vi "Camber controller May 4 2016.vi"() -> ()   [LabVIEW 2014]
uses:
  <vilib>/Instr/_visa.llb/VISA Configure Serial Port (Instr).vi
  <vilib>/Utility/file.llb/Write To Spreadsheet File (string).vi
  <vilib>/Utility/file.llb/Read From Spreadsheet File (string).vi
  Environmental Chamber LabVIEW and Instruments/Drivers and Software/keithley_6430/Keithley 6430/Public/Data/Read (Single Point).vi
  Environmental Chamber LabVIEW and Instruments/Drivers and Software/LabVIEW 8.2 Drivers/keithley_24xx/Keithley 24XX/Public/Data/Read (Single Point).vi
  Environmental Chamber LabVIEW and Instruments/Drivers and Software/keithley_24xx/Keithley 24XX/Keithley 24XX.lvlib
  Environmental Chamber LabVIEW and Instruments/Drivers and Software/keithley_6430/Keithley 6430/Keithley 6430.lvlib
panel:
  in  "Sample names 2":T1={"QCM1 sample"="aQCM2", "QCM2 sample"="aQCM2", "QCM3 sample"="aQCM3", "QCM4 sample"="aQCM4", "QCM5 sample"="aQCM5", "QCM6 sample"="aQCM6", "SRS sample"="sample_SRS", "K-2420 sample"="Keithley2420", "K-6430 sample"="Keithley6430", "K-2100 sample"="Keithley6430"}
  out "pressure chart":cluster{"pressure":dbl}(graph)
  out "K-6430 (Ohm)":cluster{"Measurement":dbl}(graph)
  out "K-2420 (Ohm)":cluster{"Resistance":sgl}(graph)
  in  "Data saving options":T2={"Save during sequence only"=TRUE, "Save now"=FALSE, "Stop program when sequence ends"=TRUE, "Delay between data points (s)"=0.0, "Experiment Notes"="", "Currently saving data"=FALSE, "Data file save path"=path ""} {"Delay between data points (s)" min=0.0 max=30.0 format="%#_13g"}
  out "Temp (C)":dbl
  in  "Set pressure parameters":T3={"valve % open"=100.0, "Desired pressure"=0.0, "Vapor sccm"=0.0, "Gas sccm"=0.0, "Valve"=enum."% Open", "Pressure Mode"=enum."Abs. pressure", "analyte partial pressure"=100.0} {"analyte partial pressure" min=0.0 max=100.0 step=5.0; "Gas sccm" min=0 max=200 step=5; "Vapor sccm" min=0 max=200 step=5; "Desired pressure" min=0.0 max=760.0 step=5.0; "valve % open" min=0.0 max=100.0 step=5.0 format="%#_2f"}
  out "Actual":T4 {"actual gas flow" format="%#_3g"; "Actual vapor flow" format="%#_3g"; "actual pressure" format="%#_3g"; "Valve position (%)" format="%#_2f"}
  out "arduino QCM plots":T5
  out "QCM Freq. (MHz)":T6 {"QCM1" format="%#_8g"; "QCM2" format="%#_8g"; "QCM3" format="%#_8g"; "QCM4" format="%#_8g"; "QCM5" format="%#_8g"; "QCM6" format="%#_8g"}
  out "Sequence\npreview":cluster{dbl[], dbl[]}[](graph)
  in  "Gate time":u16(ring)=1 items=["0.1 seconds", "1.0 seconds", "10.0 seconds"]
  out "MHz":dbl format="%.6f"
  out "QCM plot":T7(graph)
  in  "User-defined\nsequence":string[][](table) caption="Create sequence"
  out "Sequence end time":string
  in  "Run Sequence":bool
  in  "Import sequence file":bool
  in  "Save sequence":bool
  in  "Clear sequence":bool
  in  "Turbo pump\nauto on":bool=TRUE caption="Turbo pump auto on"
  out "Start Time":string
  in  "stop":bool
  in  "Clear all charts":bool
  out "appended array":dbl[](array[numeric]) caption="atm\nTorr"
  in  "rapidox O2 Sensor":bool
  in  "setnag O2 Pump":bool
  in  "Baud Rate 2":i32(ring)=2 items=["2400", "4800", "9600", "19200", "38400", "57600", "115200"]
  in  "Com Port":i32(ring) items=["Com 1", "Com 2", "Com 3", "Com 4", "Com 5", "Com 6", "COM 7", "COM 8", "COM 9", "COM 10", "COM 11", "COM 12", "com 13", "COM 14"]
  in  "Com Port 2":i32(ring) items=["Com 1", "Com 2", "Com 3", "Com 4", "Com 5", "Com 6", "COM 7", "COM 8", "COM 9", "COM 10", "COM 11", "COM 12", "com 13", "COM 14"]
  out "Waveform Chart":cluster{dbl}(graph)
  out "O2 Concentration (PPM)":dbl
  out "Waveform Chart 6":cluster{dbl}(graph)
  # "Pressure Control"
  # "Gas/Vapor Sequence"
  # "SRS QCM"
  # "Currently Unused"
  # "100%"
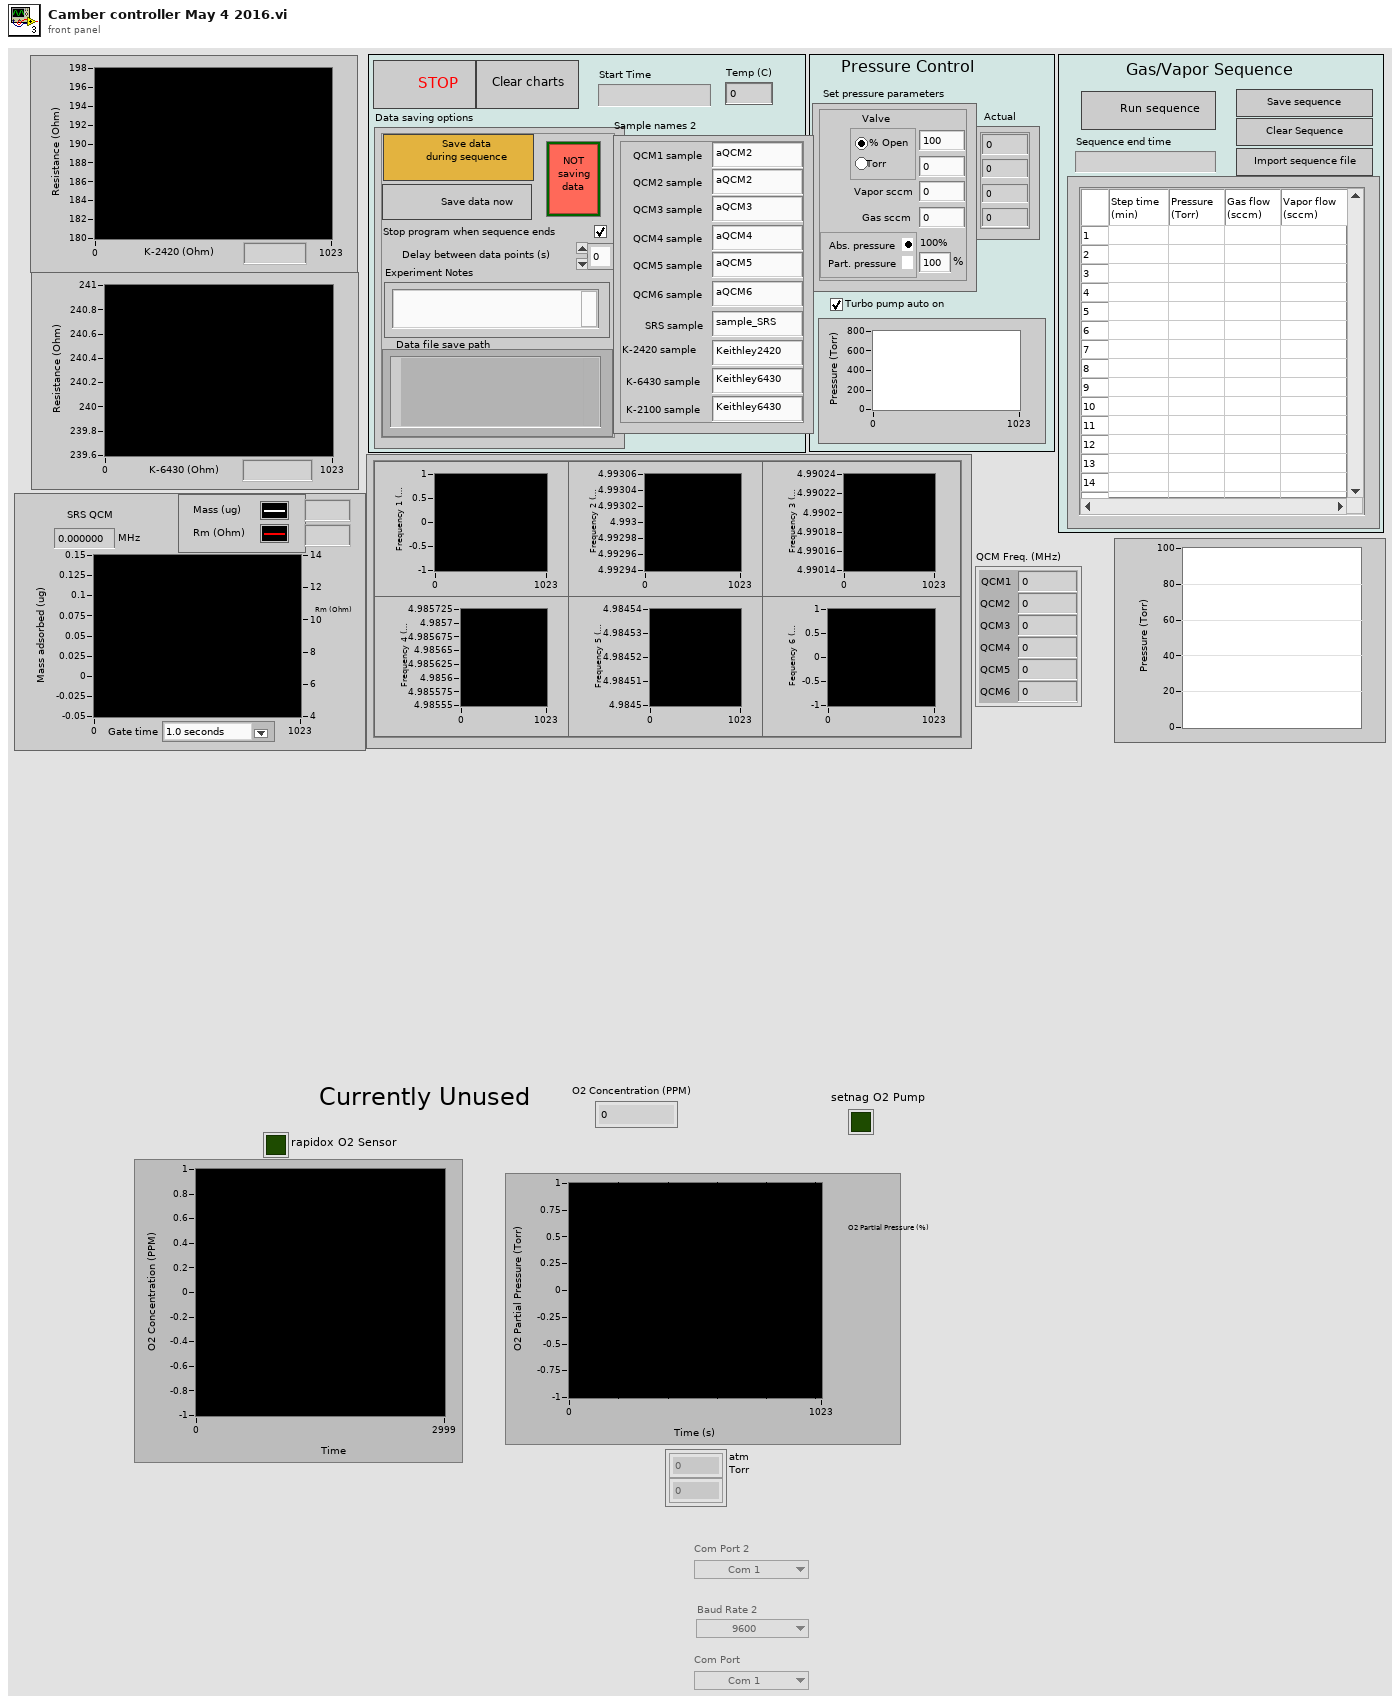
[diagram p1: front panel]
types:
  T1 = cluster{"QCM1 sample":string, "QCM2 sample":string, "QCM3 sample":string, "QCM4 sample":string, "QCM5 sample":string, "QCM6 sample":string, "SRS sample":string, "K-2420 sample":string, "K-6430 sample":string, "K-2100 sample":string}
  T2 = cluster{"Save during sequence only":bool, "Save now":bool, "Stop program when sequence ends":bool, "Delay between data points (s)":dbl, "Experiment Notes":string, "Currently saving data":bool, "Data file save path":path}
  T3 = cluster{"valve % open":dbl, "Desired pressure":dbl, "Vapor sccm":sgl, "Gas sccm":sgl, "Valve":enum32{"% Open", "Torr "}, "Pressure Mode":enum32{"Abs. pressure", " Part. pressure"}, "analyte partial pressure":dbl}
  T4 = cluster{"Valve position (%)":dbl, "actual pressure":dbl, "Actual vapor flow":dbl, "actual gas flow":dbl}
  T5 = cluster{"arduino qcm 1":dbl, "arduino qcm 2":dbl, "arduino qcm 3":dbl, "arduino qcm 4":dbl, "arduino qcm 5":dbl, "arduino qcm 6":dbl}
  T6 = cluster{"QCM1":dbl, "QCM2":dbl, "QCM3":dbl, "QCM4":dbl, "QCM5":dbl, "QCM6":dbl}
  T7 = cluster{"Numeric Control":dbl, "Resistance out":dbl}
  T8 = enum16{"open", "open or create", "create or replace", "create", "open (read only)"}
  T9 = enum16{"no parity", "odd parity", "even parity", "mark parity", "space parity"}
  T10 = enum8{"Enabled", "Disabled", "Disabled and Grayed Out"}
  T11 = cluster{"task out":refnum<k21>, "error out":errorcluster, "task out":refnum<k21>, "error out":errorcluster, "task out":refnum<k21>, "error out":errorcluster, "VISA resource name":refnum<visa-resource-name>, "error out":errorcluster}
  T12 = cluster{"task out":refnum<k21>, "error out":errorcluster, "task out":refnum<k21>, "error out":errorcluster, "task out":refnum<k21>, "error out":errorcluster, "VISA resource name out":refnum<visa-resource-name>, "error out":errorcluster}
  T13 = cluster{bool, "VISA resource name":refnum<visa-resource-name>, "error out":errorcluster}
  T14 = cluster{bool, "VISA resource name out":refnum<visa-resource-name>, "error out":errorcluster}
  T15 = cluster{"Arduino 1":refnum<visa-resource-name>, "Arduino 2":refnum<visa-resource-name>, "Arduino 3":refnum<visa-resource-name>, "Arduino 4":refnum<visa-resource-name>, "Arduino 5":refnum<visa-resource-name>, "Arduino 6":refnum<visa-resource-name>}
  T16 = cluster{"VISA resource name out":refnum<visa-resource-name>, "error out":errorcluster, "VISA resource name out":refnum<visa-resource-name>, "error out":errorcluster, "VISA resource name out":refnum<visa-resource-name>, "error out":errorcluster, "VISA resource name out":refnum<visa-resource-name>, "error out":errorcluster, "VISA resource name out":refnum<visa-resource-name>, "error out":errorcluster, "VISA resource name out":refnum<visa-resource-name>, "error out":errorcluster}
  T17 = cluster{"f":dbl, "f":dbl, "f":dbl, "f":dbl, "f":dbl, "f":dbl}
  T18 = cluster{"String":string, "String":string, "String":string}
  T19 = cluster{"Boolean":bool, "VISA resource name out":refnum<visa-resource-name>, "error out":errorcluster}
  T20 = cluster{bool, "Turbo pump\nauto on":bool, "current  step # out":i32}
  T21 = cluster{"Present (s)":dbl, "Run Sequence":bool, "Set pressure parameters":cluster{"valve % open":dbl, "Desired pressure":dbl, "Vapor sccm":sgl, "Gas sccm":sgl, "Valve":enum32{"% Open", "Torr "}, "Pressure Mode":enum32{"Abs. pressure", " Part. pressure"}, "analyte partial pressure":dbl}, "sequence end time":timestamp}
  T22 = cluster{"VISA Refnum out":refnum<visa-resource-name>, "error out":errorcluster, "VISA Refnum out":refnum<visa-resource-name>, "error out":errorcluster, "VISA Refnum out":refnum<visa-resource-name>, "error out":errorcluster, "VISA Refnum out":refnum<visa-resource-name>, "error out":errorcluster, "VISA Refnum out":refnum<visa-resource-name>, "error out":errorcluster, "VISA Refnum out":refnum<visa-resource-name>, "error out":errorcluster}
  T23 = cluster{"f":string, "f":string, "f":string, "f":string, "f":string, "f":string}
  T24 = cluster{bool, "VISA out":refnum<visa-resource-name>, "error out":errorcluster}
  T25 = cluster{"Boolean":bool, "VISA out":refnum<visa-resource-name>, "error out":errorcluster}
  T26 = cluster{"User-defined\nsequence":refnum<vi>, "Sequence end time":refnum<vi>, "Run Sequence":refnum<vi>}
  T27 = cluster{"pressure":string, "RH":string, "gas flow":string, "vapor flow":string}
  T28 = cluster{"Valve position (%)":dbl, "pressure":dbl, "vapor flow":dbl, "gas flow":dbl}
  T29 = cluster{"task out":refnum<k21>, "error out":errorcluster, "task out":refnum<k21>, "error out":errorcluster, "task out":refnum<k21>, "error out":errorcluster, "VISA Refnum out":refnum<visa-resource-name>, "error out":errorcluster}
  T30 = cluster{"sequence on?":bool, "sequence end time":timestamp, "current  step # out":i32}
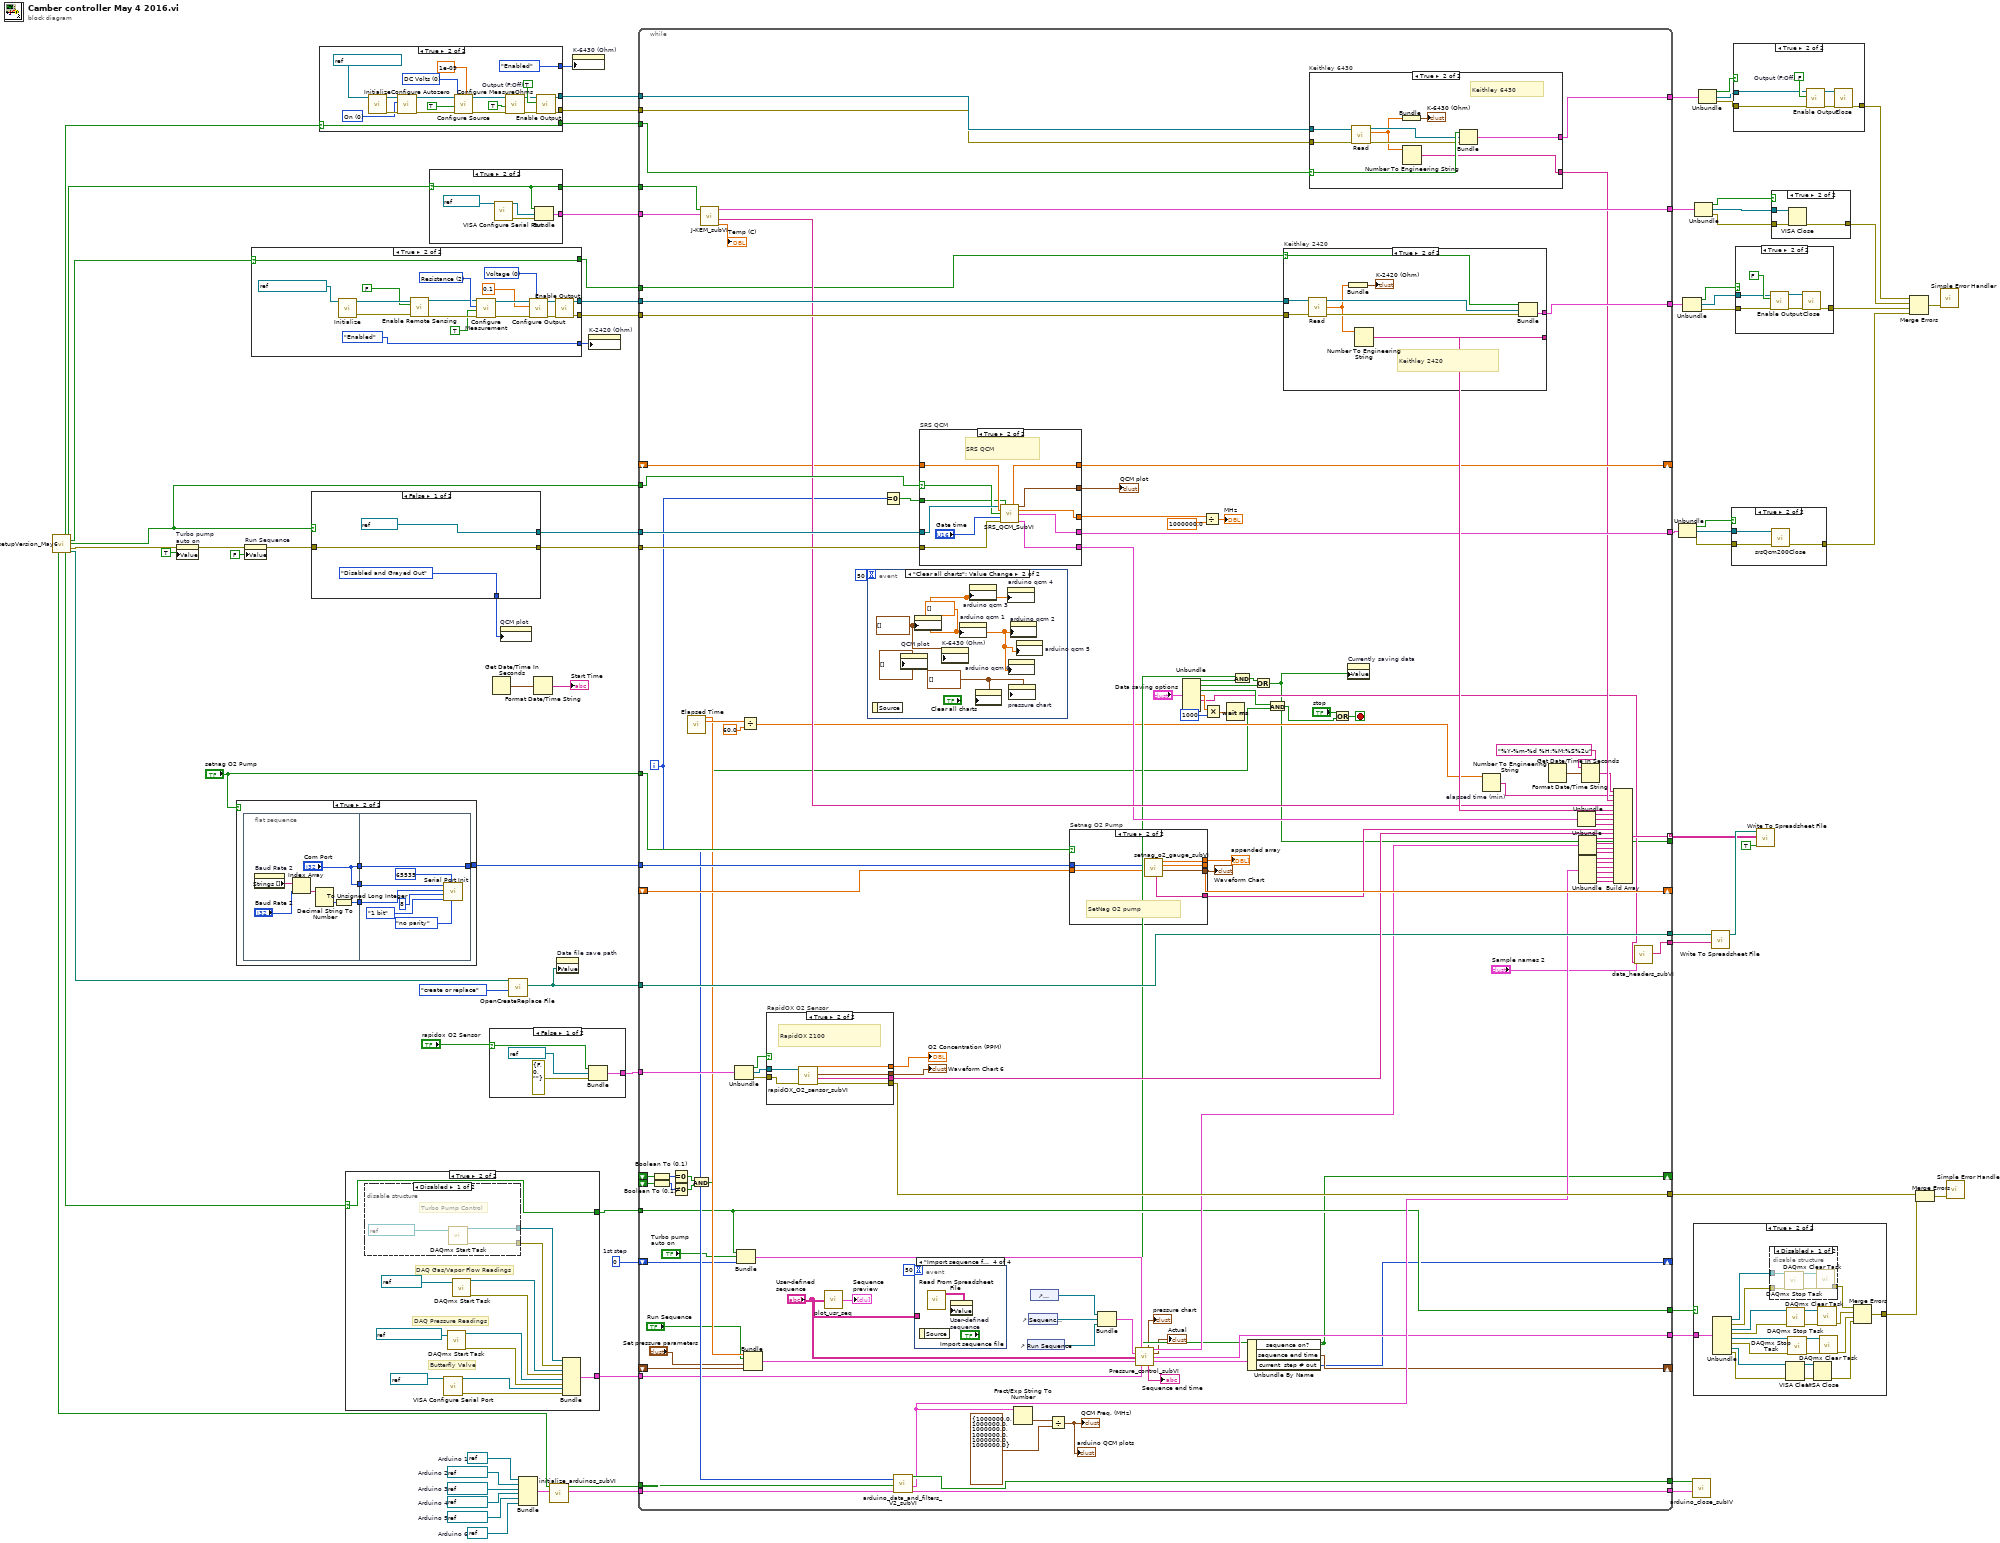
[diagram p0: block diagram]
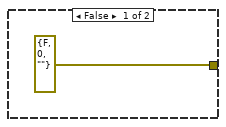
[diagram p2: hidden frame]
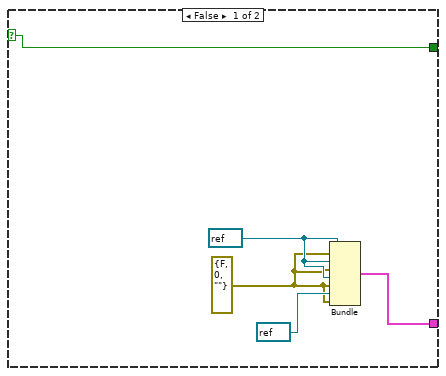
[diagram p4: hidden frame]
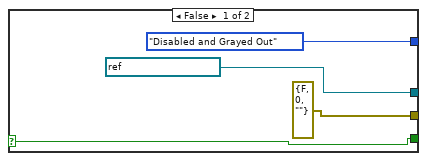
[diagram p7: hidden frame]
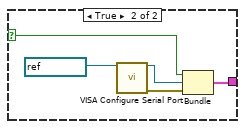
[diagram p8: hidden frame]
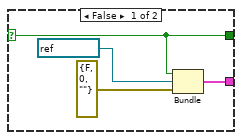
[diagram p10: hidden frame]
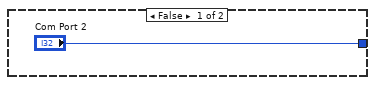
[diagram p11: hidden frame]
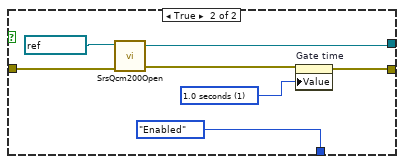
[diagram p13: hidden frame]
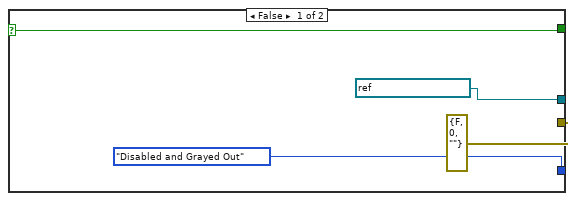
[diagram p15: hidden frame]
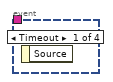
[diagram p16: hidden frame]
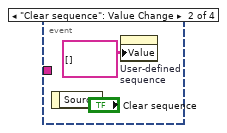
[diagram p17: hidden frame]
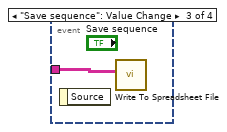
[diagram p18: hidden frame]
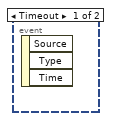
[diagram p19: hidden frame]
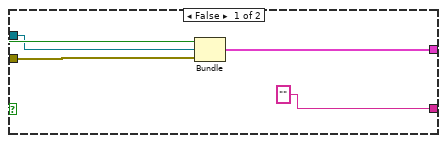
[diagram p20: hidden frame]
diagram:
  w17 = refnum<visa-resource-name> refnum  # Arduino 6
  w18 = refnum<visa-resource-name> "COM51"  # Arduino 5
  w19 = refnum<visa-resource-name> "COM50"  # Arduino 4
  w20 = refnum<visa-resource-name> "COM49"  # Arduino 3
  w21 = refnum<visa-resource-name> "COM48"  # Arduino 2
  w10 = refnum<visa-resource-name> refnum  # Arduino 1
  w37 = 0  # 1st step
  n1 = call "setupVersion_May6.vi"() -> ("Keithley 6431"=w27:bool, "J-KEM2"=w26:bool, "Keithley 2421"=w6:bool, "SRS QCM 2"=w30:bool, "error IO"=w2:errorcluster, "Arduino2"=w15:bool, "Pressure control 2"=w28:bool, "Save file path 2"=w29:path)  [unwired: 8 in]
  n2 = property on="Turbo pump\nauto on" class="Bool (strict)"(error in=w2, "Value"=TRUE ("Turbo\npump")) -> (error out=w33:errorcluster)  [unwired: 1 in, 1 out]
  n3 = case shown="True" "setnag O2 Pump" {
    tunnel: ["Com Port 2" w80] -> w72
    frame False {
    }
    frame True {
      n4 = flat-sequence {
        tunnel: ["Com Port"] -> w83
        tunnel: [w85] -> w82
        tunnel: ["Com Port"] -> w81
        tunnel: w83 -> [w91]
        tunnel: w82 -> [w90]
        tunnel: w81 -> [w92]
        tunnel: [w92] -> w80
        frame #0 {
          n5 = property on="Baud Rate 2" class="Ring (strict)"() -> ("Strings []"=w87:string[])  [unwired: 2 in, 2 out]
          n6 = Index Array(array=w87, index="Baud Rate 2") -> (element=w88:string)
          n7 = Decimal String To Number(string=w88) -> (number=w86:i32)  [unwired: 2 in, 1 out]
          n8 = To Unsigned Long Integer(number=w86) -> (unsigned 32bit integer=w85:u32)
        }
        frame #1 {
          n9 = call <vilib>:"Serial Port Init.vi"("parity"=T9."no parity", "buffer size"=u16 65535, "stop bits"=enum16{"1 bit", "1.5 bits", "2 bits"}."1 bit", "data bits"=u16 8, "baud rate"=w90, "port number"=w91) -> ()  [unwired: 1 in, 1 out]
        }
      }
    }
  }
  n10 = property on="Run Sequence" class="Bool (strict)"(error in=w33, "Value"=FALSE ("Run Sequence")) -> (error out=w35:errorcluster)  [unwired: 1 in, 1 out]
  n11 = case shown="True" w6 {
    selector: w6 -> [w97 w101]
    tunnel: [refnum<visa-resource-name> "GPIB1::24::INSTR" ("VISA resource name") w110] -> w76
    tunnel: [errorcluster {"status"=FALSE, "code"=0, "source"=""} ("error out") w105] -> w75
    tunnel: [T10."Disabled and Grayed Out" ("Disabled") T10."Enabled" ("Disabled")] -> w24
    tunnel: [w97 w101] -> w5
    frame False {
    }
    frame True {
      w112 = u16 0 items=["Voltage", "Current"] ("Source Mode  (0: Voltage)")
      w117 = u16 2 items=["Volts", "Current", "Resistance"] ("Function (0: Volts)")
      n12 = call "Initialize.vi"("VISA resource name"=refnum<visa-resource-name> "GPIB1::24::INSTR") -> ("error out"=w106:errorcluster, "VISA resource name out"=w109:refnum<visa-resource-name>)  [unwired: 9 in]
      n13 = call "Enable Remote Sensing.vi"("error in (no error)"=w106, "Enable Remote Sensing (T: Enable)"=FALSE ("4-wire?"), "VISA resource name"=w109) -> ("error out"=w107:errorcluster, "VISA resource name out"=w108:refnum<visa-resource-name>)  [unwired: 7 in]
      n14 = call "Configure Measurement.vi"("error in (no error)"=w107, "Enable Auto Range (T:Enable)"=TRUE, "Function (0: Volts)"=w117, "VISA resource name"=w108) -> ("error out"=w116:errorcluster, "VISA resource name out"=w115:refnum<visa-resource-name>)  [unwired: 6 in]
      n15 = call "Configure Output.vi"("Source Mode  (0: Voltage)"=w112, "error in (no error)"=w116, "Output Level (0)"=0.1 ("Applied Voltage (V)"), "VISA resource name"=w115) -> ("error out"=w114:errorcluster, "VISA resource name out"=w113:refnum<visa-resource-name>)  [unwired: 6 in]
      n16 = call "Enable Output.vi"("error in (no error)"=w114, "VISA resource name"=w113) -> ("error out"=w105:errorcluster, "VISA resource name out"=w110:refnum<visa-resource-name>)  [unwired: 8 in]
    }
  }
  n17 = case shown="False" w30 {
    tunnel: [refnum<visa-resource-name> "COM6" ("VISA in") w125] -> w74
    tunnel: [w120 w122] -> w73
    tunnel: w35 -> [w120 w127]
    tunnel: [T10."Disabled and Grayed Out" ("Disabled") T10."Enabled" ("Disabled")] -> w25
    frame False {
    }
    frame True {
      w124 = u16 1 items=["0.1 seconds", "1.0 seconds", "10.0 seconds"] ("Gate time")
      n18 = call "SrsQcm200Open.vi"("error in"=w127, "VISA in"=refnum<visa-resource-name> "COM6") -> ("error out"=w123:errorcluster, "VISA out"=w125:refnum<visa-resource-name>)  [unwired: 3 in]
      n19 = property on="Gate time" class="Ring (strict)"(error in=w123, "Value"=w124) -> (error out=w122:errorcluster)  [unwired: 1 in, 1 out]
    }
  }
  n20 = case shown="True" w27 {
    selector: w27 -> [w129 w133]
    tunnel: [refnum<visa-resource-name> "GPIB0::29::INSTR" ("VISA resource name") w146] -> w44
    tunnel: [errorcluster {"status"=FALSE, "code"=0, "source"=""} ("error out") w147] -> w43
    tunnel: [T10."Disabled and Grayed Out" ("Disabled") T10."Enabled" ("Disabled")] -> w23
    tunnel: [w129 w133] -> w4
    frame False {
    }
    frame True {
      w135 = u16 0 items=["DC Volts", "DC Current"] ("Source Function (0: DC Volts)")
      w142 = u16 0 items=["On", "Off", "Once"] ("Autozero  (0: On)")
      w150 = TRUE  # Output (F:Off)
      n21 = call "Initialize.vi"("VISA resource name"=refnum<visa-resource-name> "GPIB0::30::INSTR") -> ("error out"=w143:errorcluster, "VISA resource name out"=w144:refnum<visa-resource-name>)  [unwired: 4 in, 5 out]
      n22 = call "Configure Autozero.vi"("error in (no error)"=w143, "Autozero  (0: On)"=w142, "VISA resource name"=w144) -> ("error out"=w138:errorcluster, "VISA resource name out"=w140:refnum<visa-resource-name>)  [unwired: 7 in]
      n23 = call "Configure Source.vi"("I-Source Level [A]"=1e-09, "error in (no error)"=w138, "Auto Range (T:Enable)"=TRUE, "Source Function (0: DC Volts)"=w135, "VISA resource name"=w140) -> ("error out"=w137:errorcluster, "VISA resource name out"=w139:refnum<visa-resource-name>)  [unwired: 5 in]
      n24 = call "Configure MeasureOhms.vi"("error in (no error)"=w137, "Auto Range (T:Enable)"=TRUE, "VISA resource name"=w139) -> ("error out"=w151:errorcluster, "VISA resource name out"=w149:refnum<visa-resource-name>)  [unwired: 3 in, 4 out]
      n25 = call "Enable Output.vi"("error in (no error)"=w151, "Enable Output (F:Off)"=w150, "VISA resource name"=w149) -> ("error out"=w147:errorcluster, "VISA resource name out"=w146:refnum<visa-resource-name>)  [unwired: 7 out]
    }
  }
  n26 = case shown="True" w28 {
    selector: w28 -> [w152 w157]
    tunnel: [w153 w159] -> w38
    tunnel: [w152 w157] -> w3
    frame False {
      w155 = refnum<k21> refnum ("task out")
      w154 = errorcluster {"status"=FALSE, "code"=0, "source"=""} ("error out")
      n27 = Bundle("task out"=w155, "error out"=w154, "task out"=w155, "error out"=w154, "task out"=w155, "error out"=w154, "VISA resource name"=refnum<visa-resource-name> refnum, "error out"=w154) -> (w153:T11)  [unwired: 1 in]
    }
    frame True {
      # "DAQ Gas/Vapor Flow Readings"
      # "DAQ Pressure Readings"
      # "Butterfly Valve"
      n28 = disable-structure shown="Disabled" {
        disable-tunnel: [w171 _] -> w166
        disable-tunnel: [w170 _] -> w165
        frame Disabled {
          # "Turbo Pump Control"
          n29 = call <vilib>:"DAQmx Start Task.vi"("task/channels in"=refnum<k21> "TurboON") -> ("task out"=w171:refnum<k21>, "error out"=w170:errorcluster)  [unwired: 13 in]
        }
        frame Enabled {
        }
      }
      n30 = call-poly "VISA Configure Serial Port"("VISA resource name"=refnum<visa-resource-name> "COM5") -> ("VISA resource name out"=w160:refnum<visa-resource-name>, "error out"=w158:errorcluster)  [unwired: 13 in]
      n31 = call <vilib>:"DAQmx Start Task.vi"("task/channels in"=refnum<k21> "AllDaqReadings") -> ("task out"=w162:refnum<k21>, "error out"=w161:errorcluster)  [unwired: 13 in]
      n32 = call <vilib>:"DAQmx Start Task.vi"("task/channels in"=refnum<k21> "Setflow") -> ("task out"=w164:refnum<k21>, "error out"=w163:errorcluster)  [unwired: 13 in]
      n33 = Bundle("task out"=w166, "error out"=w165, "task out"=w164, "error out"=w163, "task out"=w162, "error out"=w161, "VISA resource name out"=w160, "error out"=w158) -> (w159:T12)  [unwired: 1 in]
    }
  }
  n34 = case shown="True" w26 {
    selector: w26 -> [w173 w178]
    tunnel: [w174 w179] -> w61
    tunnel: [w173 w178] -> w55
    frame False {
      n35 = Bundle(w173, "VISA resource name"=refnum<visa-resource-name> "COM3", "error out"=errorcluster {"status"=FALSE, "code"=0, "source"=""}) -> (w174:T13)  [unwired: 1 in]
    }
    frame True {
      n36 = call-poly "VISA Configure Serial Port"("VISA resource name"=refnum<visa-resource-name> "COM3") -> ("VISA resource name out"=w180:refnum<visa-resource-name>, "error out"=w177:errorcluster)  [unwired: 13 in]
      n37 = Bundle(w178, "VISA resource name out"=w180, "error out"=w177) -> (w179:T14)  [unwired: 1 in]
    }
  }
  n38 = case shown="False" "rapidox O2 Sensor" {
    selector: "rapidox O2 Sensor" -> [w182 w187]
    tunnel: [w183 w188] -> w51
    frame False {
      n39 = Bundle(w182, "VISA resource name"=refnum<visa-resource-name> "COM7", "error out"=errorcluster {"status"=FALSE, "code"=0, "source"=""}) -> (w183:T13)  [unwired: 1 in]
    }
    frame True {
      n40 = call-poly "VISA Configure Serial Port"("VISA resource name"=refnum<visa-resource-name> "COM7") -> ("VISA resource name out"=w189:refnum<visa-resource-name>, "error out"=w186:errorcluster)  [unwired: 13 in]
      n41 = Bundle(w187, "VISA resource name out"=w189, "error out"=w186) -> (w188:T14)  [unwired: 1 in]
    }
  }
  n42 = Get Date/Time In Seconds() -> (seconds since 1Jan1904=w78:timestamp)
  n43 = property on="QCM plot" class="WFChart (strict)"("DisabledEnum"=w25) -> ()  [unwired: 2 in, 2 out]
  n44 = call "OpenCreateReplace File.vi"("function (open:0)"=T8."create or replace", "file path"=w29) -> ("new file path"=w1:path)  [unwired: 6 in, 3 out]
  n45 = Bundle("Arduino 1"=w10, "Arduino 2"=w21, "Arduino 3"=w20, "Arduino 4"=w19, "Arduino 5"=w18, "Arduino 6"=w17) -> (w9:T15)  [unwired: 1 in]
  n46 = Format Date/Time String(seconds (now)=w78) -> (date/time string=→"Start Time":string)  [unwired: 2 in]
  n47 = call "initialize_arduinos_subVI.vi"("arduino 1-6 addresses"=w9, "arduinos on?"=w15) -> ("arduino 1-6 address and errors"=w14:T16, "arduinos on/off"=w16:bool)  [unwired: 8 in]
  n48 = property on="Data file save path" class="Path"("Value"=w1) -> ()  [unwired: 2 in, 2 out]
  n49 = property on="K-6430 (Ohm)" class="WFChart (strict)"("DisabledEnum"=w23) -> ()  [unwired: 2 in, 2 out]
  n50 = property on="K-2420 (Ohm)" class="WFChart (strict)"("DisabledEnum"=w24) -> ()  [unwired: 2 in, 2 out]
  n51 = while {
    shift-right: [w311] -> _
    shift-left: _ -> [w310]
    tunnel: [w281] -> w22 mode=indexing if=w192
    tunnel: w5 -> [w287]
    tunnel: w76 -> [w309]
    tunnel: w75 -> [w308]
    tunnel: w74 -> [w307]
    tunnel: w73 -> [w306]
    tunnel: w30 -> [w305]
    tunnel: "setnag O2 Pump" -> [w299]
    tunnel: w72 -> [w304]
    tunnel: [w301] -> w69
    tunnel: [w300] -> w65
    tunnel: w61 -> [w298]
    tunnel: [w297] -> w60
    tunnel: w55 -> [w295]
    tunnel: w51 -> [w293]
    tunnel: [w288] -> w31
    tunnel: [w286] -> w50
    tunnel: w1 -> [w286]
    shift-right: [w279] -> _
    shift-left: _ -> [w280]
    tunnel: w44 -> [w285]
    tunnel: w43 -> [w284]
    tunnel: [w283] -> w42
    tunnel: w3 -> [w223]
    tunnel: [w223] -> w39
    tunnel: w38 -> [w217]
    shift-right: [w219] -> _
    shift-left: w37 -> [w225]
    tunnel: [w192] -> _
    shift-right: [w220] -> _
    shift-left: _ -> [w234]
    tunnel: w16 -> [w263]
    tunnel: w14 -> [w262]
    tunnel: [w261] -> w12
    tunnel: [w260] -> w13
    tunnel: [w251] -> w11
    tunnel: [w237] -> w8
    tunnel: w4 -> [w236]
    shift-right: [w203] -> _
    shift-left: _ -> [w215]
    shift-left: _ -> [w214]
    i -> [w264]
    stop <- w199 stop-if-true
    n52 = Boolean To (0,1)(Boolean=w215) -> (0, 1=w213:i16)
    n53 = Boolean To (0,1)(Boolean=w214) -> (0, 1=w212:i16)
    n54 = Equal To 0?(x=w213) -> (x = 0?=w210:bool)
    n55 = Not Equal To 0?(x=w212) -> (x != 0?=w211:bool)
    n56 = call "Elapsed Time"() -> ("Present (s)"=w244:dbl, "Elapsed Time (s)"=w277:dbl)  [unwired: 12 in, 6 out]
    n57 = And(x=w210, y=w211) -> (x .and. y?=w197:bool)
    n58 = call "J-KEM_subVI.vi"("Address in"=w298, "J-KEM on?"=w295) -> ("Temp (C)"=→"Temp (C)":dbl, "String data out"=w296:string, "Address out"=w297:T19)  [unwired: 6 in, 1 out]
    n59 = Unbundle(w293) -> (w292:bool, "VISA resource name out"=w291:refnum<visa-resource-name>, "error out"=w290:errorcluster)
    n60 = Bundle(w223, "Turbo pump\nauto on"="Turbo pump\nauto on", "current  step # out"=w225) -> (w222:T20)  [unwired: 1 in]
    n61 = Divide(x=w277, y=60.0) -> (x/y=w201:dbl)
    n62 = Bundle("Present (s)"=w244, "Run Sequence"="Run Sequence", "Set pressure parameters"="Set pressure parameters", "sequence end time"=w234) -> (w216:T21)  [unwired: 1 in]
    n63 = case "RapidOX O2 Sensor" shown="True" w292 {
      tunnel: w291 -> [_ w343]
      tunnel: w290 -> [w336 w342]
      tunnel: ["" w341] -> w289
      tunnel: [w336 w340] -> w288
      tunnel: [0.0 w339] -> w276
      tunnel: [cluster{dbl} {0.0} w338] -> w275
      frame False {
      }
      frame True {
        # "RapidOX 2100"
        n64 = call "rapidOX_O2_sensor_subVI.vi"("error in (no error)"=w342, "VISA Refnum in"=w343) -> ("error out"=w340:errorcluster, "String"=w341:string, "Cluster"=w338:cluster{"Numeric Control":dbl}, "Numeric Control"=w339:dbl)  [unwired: 6 in]
      }
    }
    "O2 Concentration (PPM)" <- w276
    "Waveform Chart 6" <- w275
    n65 = call "plot_usr_seq.vi"("User-defined sequence"="User-defined\nsequence") -> ("Sequence Preview"=→"Sequence\npreview":cluster{dbl[], dbl[]}[])
    n66 = event shown="[1] \"Clear all charts\": Value Change" {
      selector: _ -> [_ _]
      dyn-events: _ -> [_ _]
      timeout: 50 -> [_ _]
      event Timeout {
        n67 = event-data() -> ()  [unwired: 1 in, 3 out]
      }
      event "Clear all charts": Value Change {
        w316 = cluster{dbl}[] [] ("History Data")
        w318 = cluster{"Resistance":sgl}[] [] ("History Data")
        w317 = dbl[] [] ("History Data")
        n68 = event-data() -> ()  [unwired: 1 in, 1 out]
        n69 = property on="QCM plot" class="WFChart (strict)"("History Data"=cluster{dbl, "Resistance out":dbl}[] []) -> ()  [unwired: 2 in, 2 out]
        n70 = property on="K-2420 (Ohm)" class="WFChart (strict)"("History Data"=w318) -> ()  [unwired: 2 in, 2 out]
        n71 = property on="K-6430 (Ohm)" class="WFChart (strict)"("History Data"=w318) -> ()  [unwired: 2 in, 2 out]
        n72 = property on="arduino qcm 1" class="WFChart (strict)"("History Data"=w317) -> ()  [unwired: 2 in, 2 out]
        n73 = property on="arduino qcm 3" class="WFChart (strict)"("History Data"=w317) -> ()  [unwired: 2 in, 2 out]
        n74 = property on="Waveform Chart" class="WFChart (strict)"("History Data"=w316) -> ()  [unwired: 2 in, 2 out]
        n75 = property on="arduino qcm 4" class="WFChart (strict)"("History Data"=w317) -> ()  [unwired: 2 in, 2 out]
        n76 = property on="arduino qcm 6" class="WFChart (strict)"("History Data"=w317) -> ()  [unwired: 2 in, 2 out]
        n77 = property on="pressure chart" class="WFChart (strict)"("History Data"=w316) -> ()  [unwired: 2 in, 2 out]
        n78 = property on="arduino qcm 2" class="WFChart (strict)"("History Data"=w317) -> ()  [unwired: 2 in, 2 out]
        n79 = property on="arduino qcm 5" class="WFChart (strict)"("History Data"=w317) -> ()  [unwired: 2 in, 2 out]
      }
    }
    n80 = Equal To 0?(x=w264) -> (x = 0?=w270:bool)
    n81 = call "arduino_data_and_filters_V2_subVI.vi"("loop iteration number"=w264, "arduino 1-6 address and errors"=w262, "arduinos on?"=w263) -> ("arduino 1-6 addresses and errors out"=w260:T22, "arduino 1-6 data out"=w259:T23, "arduinos on? output"=w261:bool)  [unwired: 6 in]
    n82 = event shown="[3] \"Import sequence file\": Value Change" {
      selector: _ -> [_ _ _ _]
      dyn-events: _ -> [_ _ _ _]
      timeout: 50 -> [_ _ _ _]
      tunnel: "User-defined\nsequence" -> [_ _ w314 _]
      event Timeout {
        n83 = event-data() -> ()  [unwired: 1 in, 1 out]
      }
      event "Clear sequence": Value Change {
        n84 = event-data() -> ()  [unwired: 1 in, 1 out]
        n85 = property on="User-defined\nsequence" class="Tbl (strict)"("Value"=string[][] []) -> ()  [unwired: 2 in, 2 out]
      }
      event "Save sequence": Value Change {
        n86 = event-data() -> ()  [unwired: 1 in, 1 out]
        n87 = call-poly <vilib>:"Write To Spreadsheet File.vi"("2D data"=w314) -> ()  [unwired: 7 in, 1 out]
      }
      event "Import sequence file": Value Change {
        n88 = event-data() -> ()  [unwired: 1 in, 1 out]
        n89 = call-poly <vilib>:"Read From Spreadsheet File.vi"() -> ("all rows"=w315:string[][])  [unwired: 7 in, 4 out]
        n90 = property on="User-defined\nsequence" class="Tbl (strict)"("Value"=w315) -> ()  [unwired: 2 in, 2 out]
      }
    }
    n91 = case "SRS QCM" shown="True" w305 {
      selector: w305 -> [w361 w367]
      tunnel: w307 -> [w364 w371]
      tunnel: w306 -> [w363 w372]
      tunnel: [w362 w375] -> w300
      tunnel: w280 -> [_ w374]
      tunnel: [w359 w373] -> w279
      tunnel: [T7 {"Numeric Control"=0.0, "Resistance out"=0.0} ("Cluster") w369] -> w274
      tunnel: [w359 w368] -> w250
      tunnel: w270 -> [_ w366]
      tunnel: [T18 {"String"="", "String"="", "String"=""} ("M,F,MR output cluster") w365] -> w258
      frame False {
        w359 = 0.0
        n92 = Bundle(w361, "VISA out"=w364, "error out"=w363) -> (w362:T24)  [unwired: 1 in]
      }
      frame True {
        # "SRS QCM"
        n93 = call "SRS_QCM_SubVI.vi"("VISA Refnum in"=w371, "first iteration?"=w366, "Frequency out 3"=w374, "Boolean 2"=w367, "Gate time"="Gate time", "error in (no error)"=w372) -> ("Frequency out 2"=w373:dbl, "Cluster"=w369:T7, "Frequency out"=w368:dbl, "Cluster 2"=w375:T25, "M,F,MR output cluster"=w365:T18)  [unwired: 2 in, 3 out]
      }
    }
    "QCM plot" <- w274
    n94 = Fract/Exp String To Number(string=w259) -> (number=w247:T17)  [unwired: 3 in, 1 out]
    n95 = control-ref of="Run Sequence"() -> (w227:refnum<vi>)
    n96 = control-ref of="Sequence end time"() -> (w228:refnum<vi>)
    n97 = control-ref of="User-defined\nsequence"() -> (w229:refnum<vi>)
    n98 = Divide(x=w247, y=T17 {"f"=1000000.0, "f"=1000000.0, "f"=1000000.0, "f"=1000000.0, "f"=1000000.0, "f"=1000000.0}) -> (x/y=→"QCM Freq. (MHz)" →"arduino QCM plots":T17)
    n99 = case "Setnag O2 Pump" shown="True" w299 {
      tunnel: [w379 w384] -> w311
      tunnel: w310 -> [w379 w385]
      tunnel: w304 -> [_ w383]
      tunnel: ["" w382] -> w303
      tunnel: [dbl[] [] w381] -> w273
      tunnel: [cluster{dbl} {0.0} w380] -> w272
      frame False {
      }
      frame True {
        # "SetNag O2 pump"
        n100 = call "setnag_o2_gauge_subVI.vi"("Numeric Control 3"=w385, "Com Port"=w383) -> ("Cluster"=w380:cluster{"Numeric Control":dbl}, "Numeric Control out"=w384:dbl, "Array"=w381:dbl[], "String"=w382:string)  [unwired: 6 in]
      }
    }
    "appended array" <- w273
    "Waveform Chart" <- w272
    n101 = Bundle("User-defined\nsequence"=w229, "Sequence end time"=w228, "Run Sequence"=w227) -> (w226:T26)  [unwired: 1 in]
    n102 = call "Pressure_control_subVI.vi"("press control on / turb pump on / step #"=w222, "references in"=w226, "User-defined\nsequence"="User-defined\nsequence", "output cluster"=w216, "DAQ IDs in"=w217) -> ("pressure"=→"pressure chart":cluster{"pressure":dbl}, "press/RH/gas/vapor"=w242:T27, "pressure params out"=→"Actual":T28, "DAQ IDs out"=w237:T29, "seq on/timestamp/step#"=w221:T30, "date/time string"=→"Sequence end time":string)  [unwired: 5 in]
    n103 = Unbundle("Data saving options") -> ("Save during sequence only"=w204:bool, "Save now"=w207:bool, "Stop program when sequence ends"=w198:bool, "Delay between data points (s)"=w205:dbl, "Experiment Notes"=w195:string)  [unwired: 2 out]
    n104 = Divide(x=w250, y=1000000.0) -> (x/y=→"MHz":dbl)
    n105 = Multiply(x=w205, y=u32 1000 ("x")) -> (x*y=w271:dbl)
    n106 = Wait (ms)(milliseconds to wait=w271) -> ()  [unwired: 1 out]
    n107 = Unbundle By Name(w221) -> ("sequence on?"=w203:bool, "sequence end time"=w220:timestamp, "current  step # out"=w219:i32)
    n108 = And(x=w203, y=w204) -> (x .and. y?=w202:bool)
    n109 = Or(x=w202, y=w207) -> (x .or. y?=w192:bool)
    n110 = And(x=w198, y=w197) -> (x .and. y?=w196:bool)
    n111 = case "Keithley 2420" shown="True" w287 {
      selector: w287 -> [w347 w355]
      tunnel: w309 -> [w346 w350]
      tunnel: w308 -> [w345 w349]
      tunnel: [w344 w353] -> w301
      tunnel: ["" w352] -> w302
      frame False {
        n112 = Bundle(w347, "VISA resource name out"=w346, "error out"=w345) -> (w344:T14)  [unwired: 1 in]
      }
      frame True {
        # "Keithley 2420"
        n113 = call-poly "Read.vi"("VISA resource name"=w350, "error in (no error)"=w349) -> ("VISA resource name out"=w356:refnum<visa-resource-name>, "Resistance"=w351:sgl, "error out"=w354:errorcluster)  [unwired: 7 in, 4 out]
        n114 = Bundle("Resistance"=w351) -> (→"K-2420 (Ohm)":cluster{"Resistance":sgl})  [unwired: 1 in]
        n115 = Number To Engineering String(4:w351) -> (0:w352:string)  [unwired: 3 in]
        n116 = Bundle(w355, "VISA resource name out"=w356, "error out"=w354) -> (w353:T14)  [unwired: 1 in]
      }
    }
    n117 = case "Keithley 6430" shown="True" w236 {
      selector: w236 -> [w323 w333]
      tunnel: w285 -> [w322 w330]
      tunnel: w284 -> [w321 w329]
      tunnel: ["" w332] -> w278
      tunnel: [w320 w331] -> w283
      frame False {
        n118 = Bundle(w323, "VISA resource name out"=w322, "error out"=w321) -> (w320:T14)  [unwired: 1 in]
      }
      frame True {
        # "Keithley 6430"
        n119 = call-poly "Read.vi"("error in (no error)"=w329, "VISA resource name"=w330) -> ("error out"=w328:errorcluster, "Measurement"=w326:dbl, "VISA resource name out"=w327:refnum<visa-resource-name>)  [unwired: 1 in, 6 out]
        n120 = Bundle("Measurement"=w326) -> (→"K-6430 (Ohm)":cluster{"Measurement":dbl})  [unwired: 1 in]
        n121 = Number To Engineering String(4:w326) -> (0:w332:string)  [unwired: 3 in]
        n122 = Bundle(w333, "VISA resource name out"=w327, "error out"=w328) -> (w331:T14)  [unwired: 1 in]
      }
    }
    n123 = Or(x="stop", y=w196) -> (x .or. y?=w199:bool)
    n124 = property on="Currently saving data" class="Bool (strict)"("Value"=w192) -> ()  [unwired: 2 in, 2 out]
    n125 = Number To Engineering String "elapsed time (min)"(4:w201) -> (0:w208:string)  [unwired: 3 in]
    n126 = Get Date/Time In Seconds() -> (seconds since 1Jan1904=w312:timestamp)
    n127 = Unbundle(w258) -> ("String"=w268:string, "String"=w267:string, "String"=w266:string)
    n128 = Unbundle(w242) -> ("pressure"=w241:string, "RH"=w240:string, "gas flow"=w239:string, "vapor flow"=w238:string)
    n129 = Unbundle ("arduino 1-6")(w259) -> ("f"=w257:string, "f"=w256:string, "f"=w255:string, "f"=w254:string, "f"=w253:string, "f"=w252:string)
    n130 = Format Date/Time String(time format string (%c)="%Y-%m-%d %H:%M:%S%2u", seconds (now)=w312) -> (date/time string=w265:string)  [unwired: 1 in]
    n131 = Build Array(w265, w208, w278, w296, w302, w268, w267, w266, w303, w289, w241, w240, w239, w238, w257, w256, w255, w254, w253, w252) -> (w281:string[])
    n132 = call "data_headers_subVI.vi"("Experiment Notes"=w195, "Sample names"="Sample names 2") -> ("data headers"=w251:string[])  [unwired: 9 in]
  }
  n133 = Unbundle(w65) -> ("Boolean"=w64:bool, "VISA out"=w63:refnum<visa-resource-name>, "error out"=w62:errorcluster)
  n134 = Unbundle(w69) -> (w68:bool, "VISA resource name out"=w67:refnum<visa-resource-name>, "error out"=w66:errorcluster)
  n135 = call "arduino_close_subIV.vi"("arduino 1-6 addresses and errors out"=w13, "arduinos on?"=w12) -> ()  [unwired: 10 in]
  n136 = case shown="True" w39 {
    tunnel: w8 -> [_ w400]
    tunnel: [errorcluster {"status"=FALSE, "code"=0, "source"=""} ("error out") w387] -> w7
    frame False {
    }
    frame True {
      n137 = Unbundle(w400) -> ("task out"=w399:refnum<k21>, "error out"=w398:errorcluster, "task out"=w397:refnum<k21>, "error out"=w396:errorcluster, "task out"=w395:refnum<k21>, "error out"=w394:errorcluster, "VISA Refnum out"=w393:refnum<visa-resource-name>, "error out"=w392:errorcluster)
      n138 = disable-structure shown="Disabled" {
        disable-tunnel: [w409 _] -> w391
        disable-tunnel: w399 -> [w408 _]
        disable-tunnel: w398 -> [w407 _]
        frame Disabled {
          n139 = call <vilib>:"DAQmx Stop Task.vi"("task/channels in"=w408, "error in"=w407) -> ("task out"=w410:refnum<k21>, "error out"=w411:errorcluster)  [unwired: 12 in]
          n140 = call <vilib>:"DAQmx Clear Task.vi"("task in"=w410, "error in"=w411) -> ("error out"=w409:errorcluster)  [unwired: 13 in]
        }
        frame Enabled {
        }
      }
      n141 = VISA Clear(VISA resource name=w393, error in (no error)=w392) -> (VISA resource name out=w402:refnum<visa-resource-name>, error out=w401:errorcluster)
      n142 = call <vilib>:"DAQmx Stop Task.vi"("task/channels in"=w397, "error in"=w396) -> ("task out"=w404:refnum<k21>, "error out"=w403:errorcluster)  [unwired: 12 in]
      n143 = call <vilib>:"DAQmx Stop Task.vi"("task/channels in"=w395, "error in"=w394) -> ("task out"=w405:refnum<k21>, "error out"=w406:errorcluster)  [unwired: 12 in]
      n144 = VISA Close(VISA resource name=w402, error in (no error)=w401) -> (error out=w388:errorcluster)
      n145 = call <vilib>:"DAQmx Clear Task.vi"("task in"=w404, "error in"=w403) -> ("error out"=w390:errorcluster)  [unwired: 13 in]
      n146 = call <vilib>:"DAQmx Clear Task.vi"("task in"=w405, "error in"=w406) -> ("error out"=w389:errorcluster)  [unwired: 13 in]
      n147 = Merge Errors(w391, w390, w389, w388) -> (w387:errorcluster)
    }
  }
  n148 = Unbundle(w60) -> ("Boolean"=w59:bool, "VISA resource name out"=w58:refnum<visa-resource-name>, "error out"=w57:errorcluster)
  n149 = Unbundle(w42) -> (w47:bool, "VISA resource name out"=w46:refnum<visa-resource-name>, "error out"=w45:errorcluster)
  n150 = call-poly <vilib>:"Write To Spreadsheet File.vi"("1D data"=w11, "file path (dialog if empty)"=w50) -> ("new file path (Not A Path if cancelled)"=w54:path)  [unwired: 6 in]
  n151 = case shown="True" w64 {
    tunnel: w62 -> [w412 w415]
    tunnel: [w412 w414] -> w71
    tunnel: w63 -> [_ w413]
    frame False {
    }
    frame True {
      n152 = call "srsQcm200Close.vi"("error in"=w415, "Visa in"=w413) -> ("error out"=w414:errorcluster)  [unwired: 3 in]
    }
  }
  n153 = case shown="True" w47 {
    tunnel: w46 -> [_ w418]
    tunnel: w45 -> [w416 w417]
    tunnel: [w416 w419] -> w41
    frame False {
    }
    frame True {
      w422 = FALSE  # Output (F:Off)
      n154 = call "Enable Output.vi"("error in (no error)"=w417, "Enable Output (F:Off)"=w422, "VISA resource name"=w418) -> ("error out"=w420:errorcluster, "VISA resource name out"=w421:refnum<visa-resource-name>)  [unwired: 7 out]
      n155 = call "Close.vi"("error in (no error)"=w420, "VISA resource name"=w421) -> ("error out"=w419:errorcluster)  [unwired: 9 out]
    }
  }
  n156 = case shown="True" w68 {
    tunnel: w67 -> [_ w426]
    tunnel: w66 -> [w423 w425]
    tunnel: [w423 w424] -> w70
    frame False {
    }
    frame True {
      n157 = call "Enable Output.vi"("error in (no error)"=w425, "Enable Output (T: Enable)"=FALSE, "VISA resource name"=w426) -> ("error out"=w427:errorcluster, "VISA resource name out"=w429:refnum<visa-resource-name>)  [unwired: 7 in]
      n158 = call "Close.vi"("error in (no error)"=w427, "VISA resource name"=w429) -> ("error out"=w424:errorcluster)  [unwired: 9 in]
    }
  }
  n159 = call-poly <vilib>:"Write To Spreadsheet File.vi"("append to file? (new file:F)"=TRUE, "2D data"=w22, "file path (dialog if empty)"=w54) -> ()  [unwired: 5 in, 1 out]
  n160 = case shown="True" w59 {
    tunnel: w58 -> [_ w433]
    tunnel: w57 -> [w430 w432]
    tunnel: [w430 w431] -> w56
    frame False {
    }
    frame True {
      n161 = VISA Close(VISA resource name=w433, error in (no error)=w432) -> (error out=w431:errorcluster)
    }
  }
  n162 = Merge Errors(w41, w56, w70, w71) -> (w77:errorcluster)
  n163 = Merge Errors(w31, w7) -> (w32:errorcluster)
  n164 = call <vilib>:"Simple Error Handler.vi"("error in (no error)"=w77) -> ()  [unwired: 4 in, 5 out]
  n165 = call <vilib>:"Simple Error Handler.vi"("error in (no error)"=w32) -> ()  [unwired: 4 in, 5 out]
